vi "量测结果汇总.vi"(4 "显示坐标":cluster{dbl, "Numeric":dbl}[](array[cluster])=[{300.0, "Numeric"=200.0}, {300.0, "Numeric"=400.0}, {300.0, "Numeric"=600.0}, {300.0, "Numeric"=800.0}, {300.0, "Numeric"=1000.0}, {300.0, "Numeric"=1200.0}, {300.0, "Numeric"=1400.0}], 5 "Font, Size & Style":T1={"Desired Font (Application)"=enum."User-specified Font", "[User-specified Font]"={"Font Name"="", "Size"=120, "Strikeout?"=FALSE, "Italic?"=FALSE, "Underline?"=FALSE, "Outline?"=FALSE, "Shadow?"=FALSE, "Bold?"=FALSE, "Rotation Angle"=0.0}, "Horizontal Alignment"=0, "Vertical Alignment"=0} {"Horizontal Alignment" items=["Left", "Center", "Right"]; "Vertical Alignment" items=["Bottom", "Top", "Baseline"]}, 6 "选项":enum16{"相机1", "相机2", "相机3", "相机4"}(ring), 8 "量测数据1维":dbl[](array[numeric]), 9 "Img in":T3) -> (1 "存档数据":T2, 2 "结果":bool, 3 "ImgOut":T3)   [LabVIEW 2014]
doc: "量测项目数值：每行代表单个量测项目的数值有多少行就有多少个量测项目\n数量：每个量测项目的量测数值的数量\n”数量“ 数组大小与“量测项目数值”的行数一样"
uses:
  <vilib>/vision/Image Controls.llb/IMAQ Image.ctl
  Global.vi
panel:
  out "数组":dbl[](array[numeric])
  out "当前零件型号":string
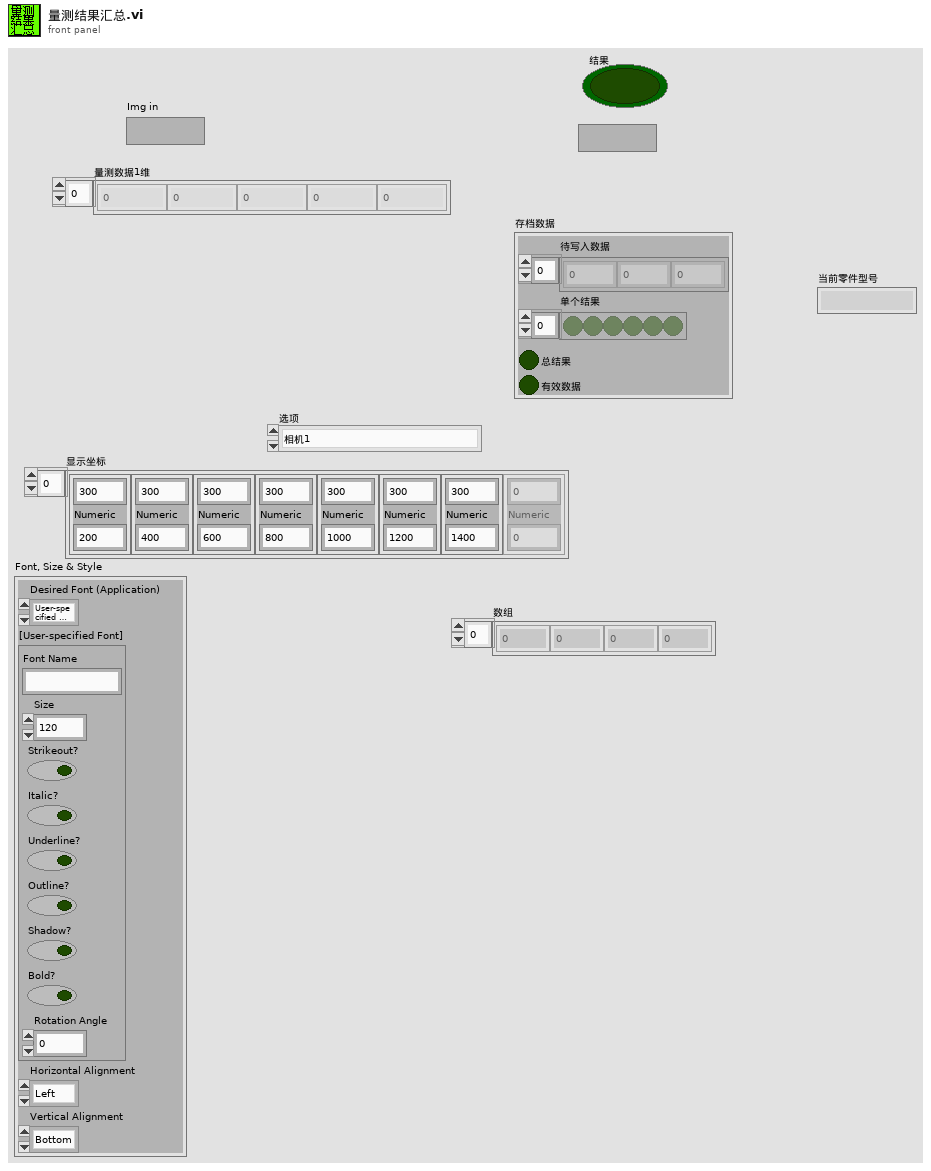
[diagram p1: front panel]
types:
  T1 = cluster{"Desired Font (Application)":enum16{"User-specified Font", "Application Font", "System Font", "Dialog Font"}, "[User-specified Font]":cluster{"Font Name":string, "Size":i16, "Strikeout?":bool, "Italic?":bool, "Underline?":bool, "Outline?":bool, "Shadow?":bool, "Bold?":bool, "Rotation Angle":dbl}, "Horizontal Alignment":i16, "Vertical Alignment":i16}
  T2 = typedef "控件-存档数据和结果.ctl" = cluster{"待写入数据":dbl[], "单个结果":bool[], "总结果":bool, "有效数据":bool}
  T3 = typedef "IMAQ Image.ctl" = refnum<image>
  T4 = typedef "OtherSpec.ctl" = cluster{"其它勾选类规格":T5, "其它数据类规格":T6, "相机名称":T7, "参数":cluster{"Mark1曝光时间":i32, "Mark2曝光时间":i32, "二维码曝光时间":i32}}
  T5 = typedef "其它勾选类规格.ctl" = cluster{"保存NG图片":bool, "保存OK图片":bool, "保存数据":bool, "开机默认开启监控摄像头":bool}
  T6 = typedef "其他数据类规格.ctl" = cluster{"相机1像素-毫米换算系数":dbl, "相机2像素-毫米换算系数":dbl, "D盘剩余空间预警(G)":dbl, "视频最长录制时间(秒)":dbl}
  T7 = typedef "相机名称品牌使用状态.ctl" = cluster{"相机1名称":T8, "相机2名称":T8, "Cam1启用":bool, "Cam2启用":bool, "Basler1":bool, "Basler2":bool}
  T8 = typedef "IMAQdx.ctl" = refnum<k21>
  T9 = typedef "ModeEditeControl.ctl" = cluster{"AllModelFold":path, "AllModelNamePath":path, "所有零件型号":string[], "当前零件型号":string, "所有建立零件信息":string[][], "当前零件序号":i32, "当前产品信息":T10}
  T10 = typedef "ModelInfo.ctl" = cluster{"产品型号":string, "二维码拍照":u32, "Mark点拍照":u32}
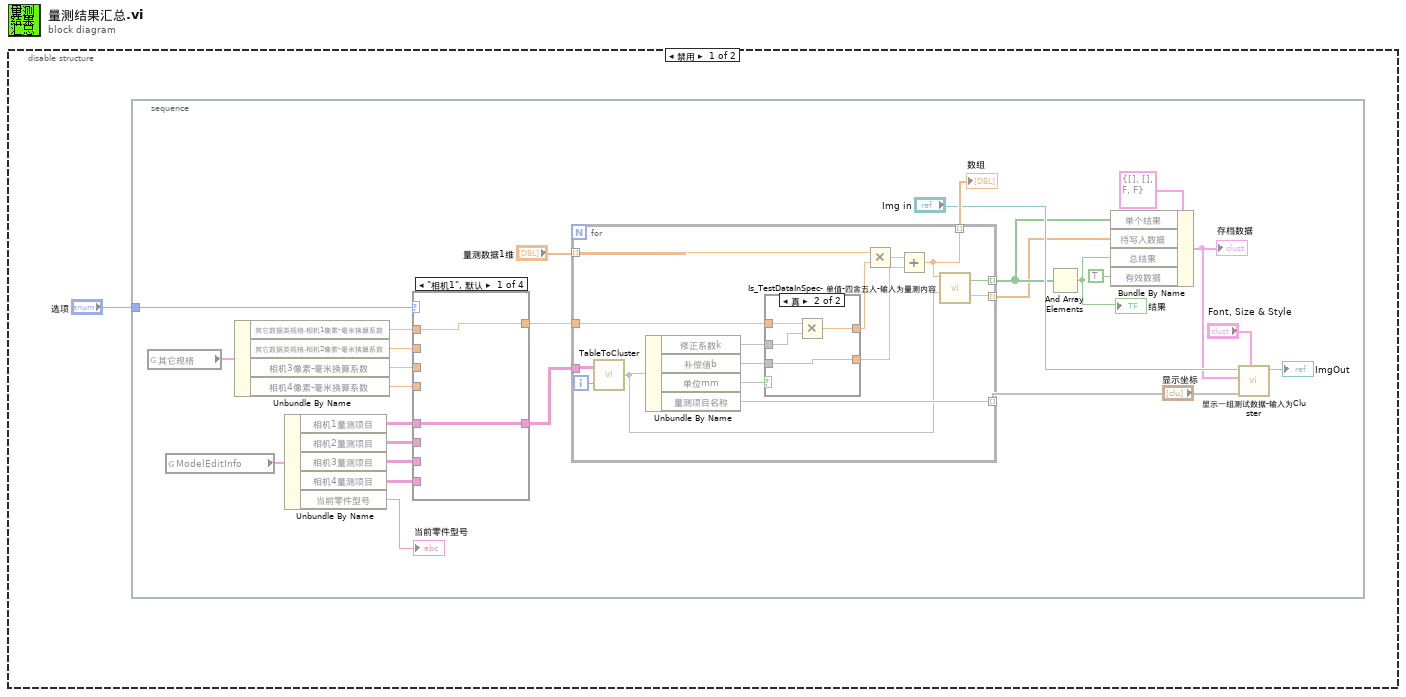
[diagram p0: block diagram]
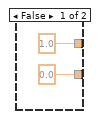
[diagram p5: hidden frame]
diagram:
  n1 = disable-structure shown="禁用" {
    frame Disabled {
      n2 = stacked-sequence {
        tunnel: "选项" -> [w20]
        frame #0 {
          n3 = global read "Global.vi" "其它规格"() -> (w14:T4)
          n4 = global read "Global.vi" "ModelEditInfo"() -> (w15:T9)
          n5 = Unbundle By Name(w14) -> ("其它数据类规格.相机1像素-毫米换算系数"=w23:dbl, "其它数据类规格.相机2像素-毫米换算系数"=w22:dbl, "相机3像素-毫米换算系数"=w21:dbl, "相机4像素-毫米换算系数"=w13:dbl)
          n6 = Unbundle By Name(w15) -> ("相机1量测项目"=w27:string[][], "相机2量测项目"=w26:string[][], "相机3量测项目"=w25:string[][], "相机4量测项目"=w24:string[][], "当前零件型号"=→"当前零件型号":string)
          n7 = case shown="\"相机1\", 默认" w20 {
            tunnel: [w30 w32 w34 w36] -> w17
            tunnel: [w29 w31 w33 w35] -> w28
            tunnel: w27 -> [w30 _ _ _]
            tunnel: w26 -> [_ w32 _ _]
            tunnel: w25 -> [_ _ w34 _]
            tunnel: w24 -> [_ _ _ w36]
            tunnel: w23 -> [w29 _ _ _]
            tunnel: w22 -> [_ w31 _ _]
            tunnel: w21 -> [_ _ w33 _]
            tunnel: w13 -> [_ _ _ w35]
            frame "相机1", Default {
            }
            frame "相机2" {
            }
            frame "相机3" {
            }
            frame "相机4" {
            }
          }
          n8 = for {
            tunnel: w28 -> [w51]
            tunnel: "量测数据1维" -> [w41] mode=indexing
            tunnel: [w42] -> w10 mode=indexing
            tunnel: w17 -> [w40]
            tunnel: [w44] -> w5 mode=indexing
            tunnel: [w39] -> w16 mode=indexing
            tunnel: [w38] -> w9 mode=indexing
            i -> [w43]
            n9 = call "TableToCluster.vi"(1:w43, 2:w40) -> (0:w37)
            n10 = Unbundle By Name(w37) -> ("修正系数k"=w48, "补偿值b"=w45, "单位mm"=w47, "量测项目名称"=w44)
            n11 = case shown="真" w47 {
              tunnel: [1.0 w56] -> w50
              tunnel: w51 -> [_ w57]
              tunnel: w48 -> [_ w54]
              tunnel: [0.0 w55] -> w46
              tunnel: w45 -> [_ w55]
              frame False {
              }
              frame True {
                n12 = Multiply(x=w57, y=w54) -> (x*y=w56:dbl)
              }
            }
            n13 = Multiply(x=w41, y=w50) -> (x*y=w49:dbl)
            n14 = Add(x=w49, y=w46) -> (x+y=w39:dbl)
            n15 = call "Is_TestDataInSpec- 单值-四舍五入-输入为量测内容.vi"("量测内容"=w37, "数值"=w39) -> ("进位舍位后值"=w38:dbl, "在规格内"=w42:bool)  [unwired: 2 in]
          }
          "数组" <- w16
          n16 = And Array Elements(Boolean array=w10) -> (logical AND=w8:bool)
          "结果" <- w8
          n17 = Bundle By Name(cluster=T2 {"待写入数据"=[], "单个结果"=[], "总结果"=FALSE, "有效数据"=FALSE} ("存档数据和结果"), "单个结果"=w10, "待写入数据"=w9, "总结果"=w8, "有效数据"=TRUE) -> (w6:T2)
          "存档数据" <- w6
          n18 = call "显示一组测试数据-输入为Cluster.vi"("量测项名称"=w5, "Font, Size & Style"="Font, Size & Style", "显示坐标"="显示坐标", "存档数据"=w6, "Img"="Img in") -> ("Img out"=→"ImgOut":T3)  [unwired: 6 in]
        }
      }
    }
    frame Enabled {
    }
  }
